vi "PicoScope2000Errorhandler.vi"(0 "Handle in":i16, 1 "API function":string, 2 "Return":i16, 3 "error in (no error)":errorcluster) -> (7 "Handle out":i16, 10 "error out":errorcluster)   [LabVIEW 2009]
uses:
  ps2000.dll
  PS2000 error codes.ctl
panel:
  in  "enPS2000Error":T1
  out "PS2000_ERROR":string
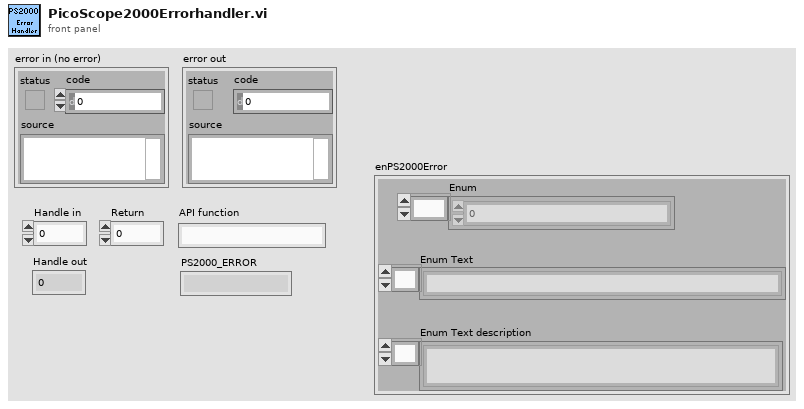
[diagram p1: front panel]
types:
  T1 = typedef "PS2000 error codes.ctl" = cluster{"Enum":u32[], "Enum Text":string[], "Enum Text description":string[]}
  T2 = enum16{"PS2000_OK", "PS2000_MAX_UNITS_OPENED", "PS2000_MEM_FAIL", "PS2000_NOT_FOUND", "PS2000_FW_FAIL", "PS2000_NOT_RESPONDING", "PS2000_CONFIG_FAIL", "PS2000_OS_NOT_SUPPORTED"}
  T3 = enum16{"Left Button", "Center Button", "Right Button", "Window Close"}
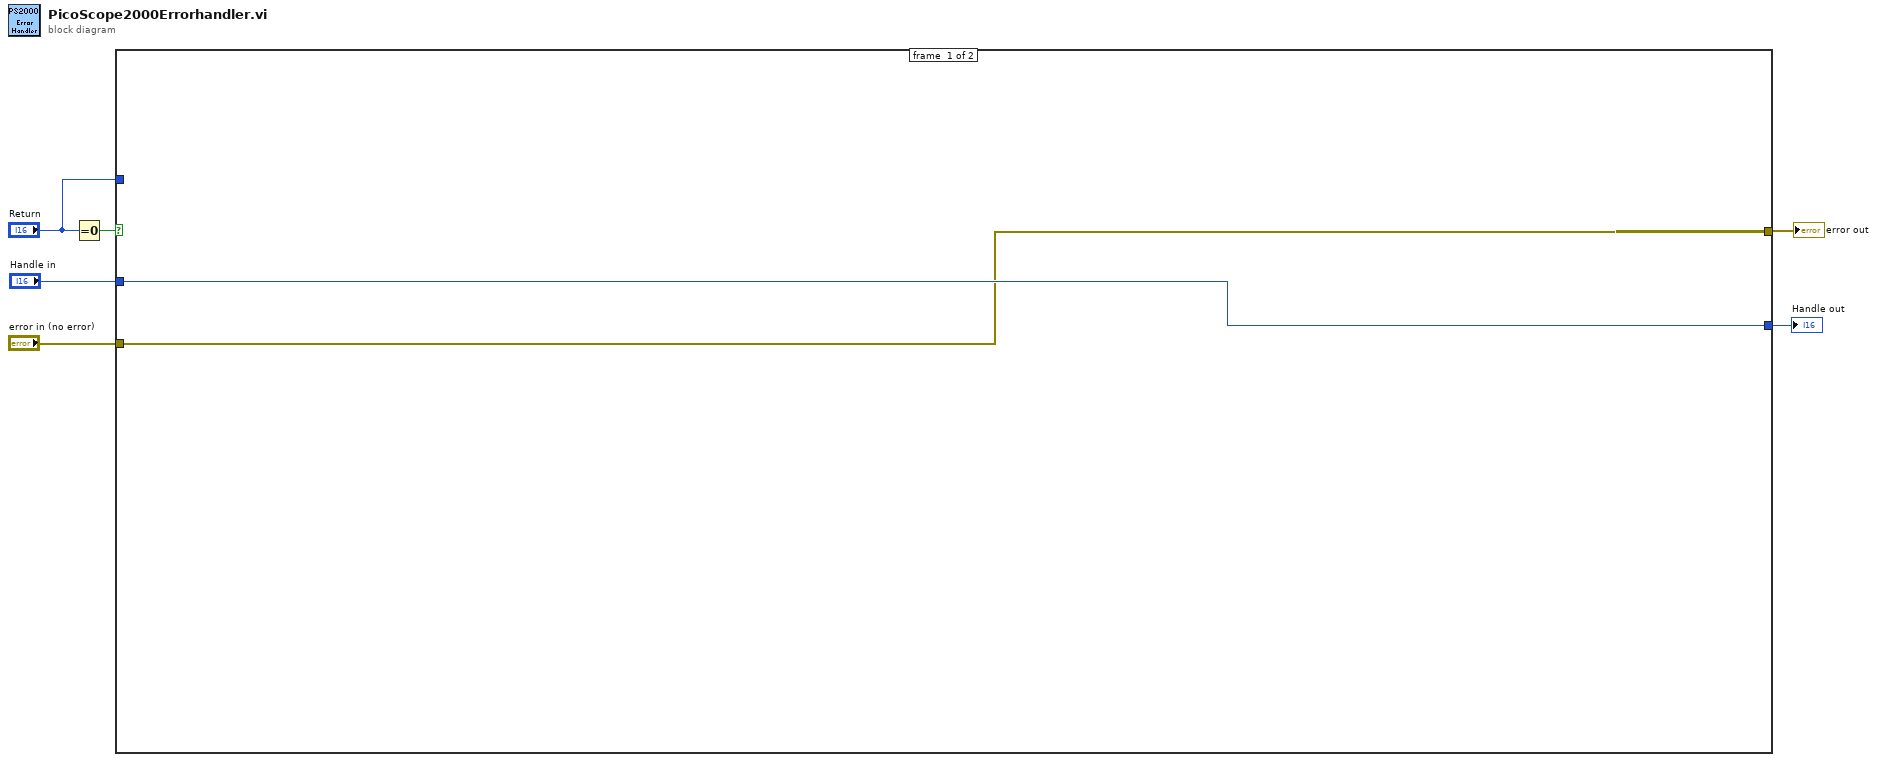
[diagram p0: block diagram]
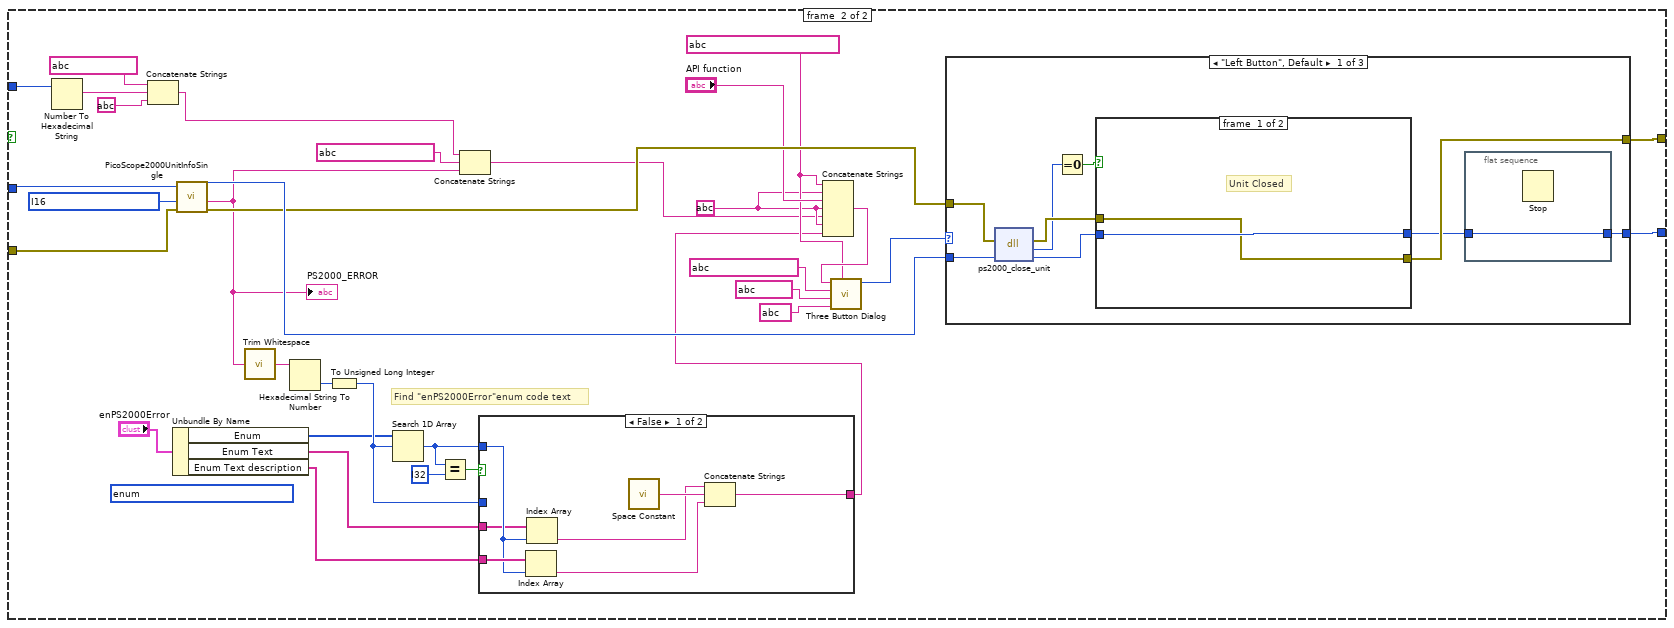
[diagram p2: hidden frame]
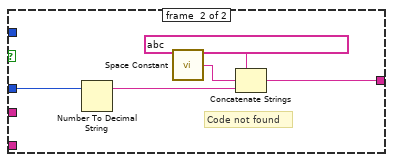
[diagram p3: hidden frame]
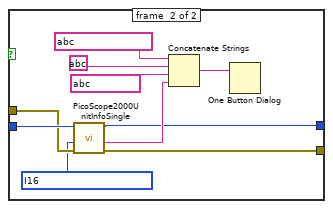
[diagram p4: hidden frame]
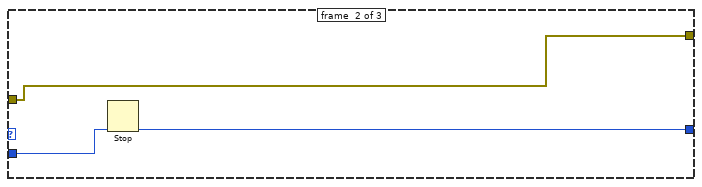
[diagram p5: hidden frame]
diagram:
  n1 = Equal To 0?(x="Return") -> (x = 0?=w5:bool)
  n2 = case shown="True" w5 {
    tunnel: "Handle in" -> [w8 w42]
    tunnel: [w8 w41] -> w4
    tunnel: "error in (no error)" -> [w7 w40]
    tunnel: [w7 w39] -> w2
    tunnel: "Return" -> [_ w17]
    frame #0 {
    }
    frame #1 {
      w28 = string ?
      w29 = string ?
      w38 = i16 ? items=["PS2000_ERROR_CODE"]
      (unwired) T2 ?
      # "Find \"enPS2000Error\"enum code text"
      n3 = Number To Hexadecimal String(2:w17) -> (0:w16:string)  [unwired: 1 in]
      n4 = Concatenate Strings(string ? ("string"), w16, string ?) -> (w13:string)
      n5 = Unbundle By Name("enPS2000Error") -> ("Enum"=w20:u32[], "Enum Text"=w19:string[], "Enum Text description"=w24:string[])
      n6 = call "PicoScope2000UnitInfoSingle.vi"("error in (no error)"=w40, "info Enum"=w38, "Handle in"=w42) -> ("error out"=w36:errorcluster, "trimmed string"=w10:string, "handle out"=w37:i16)  [unwired: 6 in]
      "PS2000_ERROR" <- w10
      n7 = call <vilib>:"Trim Whitespace.vi"("string"=w10) -> ("trimmed string"=w23:string)  [unwired: 1 in]
      n8 = Hexadecimal String To Number(string=w23) -> (number=w22:u32)  [unwired: 2 in, 1 out]
      n9 = To Unsigned Long Integer(number=w22) -> (unsigned 32bit integer=w21:u32)
      n10 = Search 1D Array(1D array=w20, element=w21) -> (index of element=w26:i32)  [unwired: 1 in]
      n11 = Equal?(x=w26, y=i32 ?) -> (x = y?=w27:bool)
      n12 = Concatenate Strings(w13, string ? ("string"), w10) -> (w12:string)
      n13 = case shown="False" w27 {
        tunnel: w26 -> [w48 _]
        tunnel: w21 -> [_ w54]
        tunnel: [w45 w53] -> w9
        tunnel: w24 -> [w49 _]
        tunnel: w19 -> [w47 _]
        frame #0 {
          n14 = Index Array(array=w49, index=w48) -> (element=w43:string)
          n15 = Index Array(array=w47, index=w48) -> (element=w44:string)
          n16 = call <vilib>:"Space Constant.vi"() -> ("String"=w46:string)
          n17 = Concatenate Strings(w44, w46, w43) -> (w45:string)
        }
        frame #1 {
          # "Code not found"
          n18 = Number To Decimal String(number=w54) -> (decimal integer string=w51:string)  [unwired: 1 in]
          n19 = call <vilib>:"Space Constant.vi"() -> ("String"=w52:string)
          n20 = Concatenate Strings(string ? ("String"), w52, w51) -> (w53:string)
        }
      }
      n21 = Concatenate Strings(w29, w28, "API function", w28, w12, w28, w9) -> (w31:string)
      n22 = call <vilib>:"Three Button Dialog.vi"("Window Title (\"\")"=w29, "Right Button Text (\"Cancel\")"=string ? ("Right Button Text (\"Cancel\")"), "Center Button Text (\"No\")"=string ? ("Center Button Text (\"No\")"), "Left Button Text (\"Yes\")"=string ? ("Left Button Text (\"Yes\")"), "message"=w31) -> ("Which Button?"=w32:T3)  [unwired: 6 in]
      n23 = case shown="\"Left Button\", Default" w32 {
        tunnel: w37 -> [w61 w78 w80]
        tunnel: [w63 w78 w80] -> w41
        tunnel: w36 -> [w62 w77 w79]
        tunnel: [w57 w77 w79] -> w39
        frame #0 {
          n24 = dll-call lib="ps2000.dll" fn="ps2000_close_unit" ("ps3000.dll:_ps3000_open_unit@0")(error in=w62, "handle"=w61) -> (error out=w58:errorcluster, "return"=w55:i16, "handle"=w59:i16)  [unwired: 2 in, 1 out]
          n25 = Equal To 0?(x=w55) -> (x = 0?=w60:bool)
          n26 = case shown="True" w60 {
            tunnel: w59 -> [w65 w75]
            tunnel: w58 -> [w64 w74]
            tunnel: [w64 w73] -> w57
            tunnel: [w65 w67] -> w56
            frame #0 {
              # "Unit Closed"
            }
            frame #1 {
              w66 = i16 ? items=["PS2000_ERROR_CODE"]
              n27 = call "PicoScope2000UnitInfoSingle.vi"("error in (no error)"=w74, "info Enum"=w66, "Handle in"=w75) -> ("error out"=w73:errorcluster, "trimmed string"=w68:string, "handle out"=w67:i16)  [unwired: 6 in]
              n28 = Concatenate Strings(string ? ("string"), string ?, string ? ("string"), w68) -> (w72:string)
              n29 = One Button Dialog(message=w72) -> ()  [unwired: 1 in, 1 out]
            }
          }
          n30 = flat-sequence {
            tunnel: w56 -> [w76]
            tunnel: [w76] -> w63
            frame #0 {
              n31 = Stop() -> ()  [unwired: 1 in]
            }
          }
        }
        frame #1 {
          n32 = Stop() -> ()  [unwired: 1 in]
        }
        frame #2 {
        }
      }
    }
  }
  "Handle out" <- w4
  "error out" <- w2
